vi "Assemble_Vision_Judge.vi"(11 "D3006 R合蓋結果":bool[](array[boolean])) -> (2 "結果":string)   [LabVIEW 2019]
panel:
  out "appended array":bool[](array[boolean])
  # "1. 無定位點\n2. 無塑膠件\n3. 無旋開\n4. 無限位\n5. 保留一\n6. 保留二"
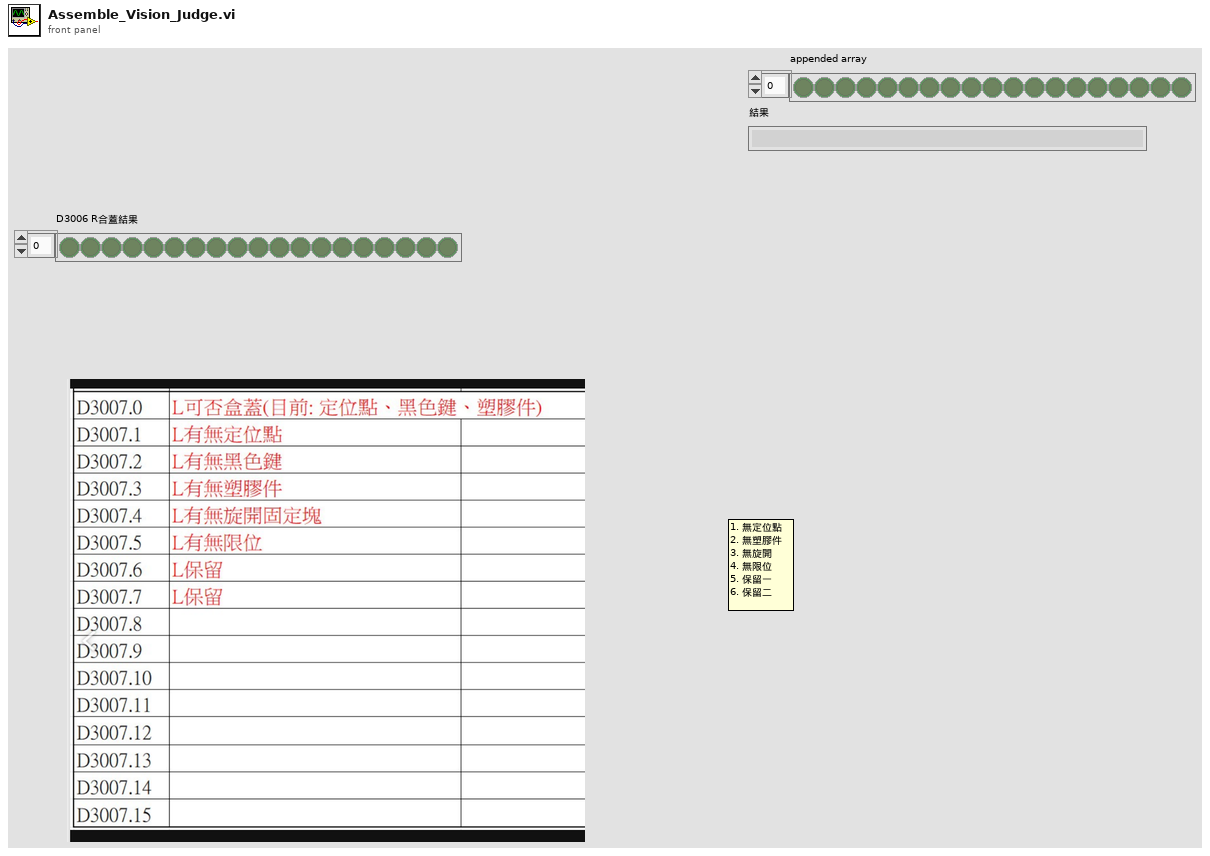
[diagram p1: front panel]
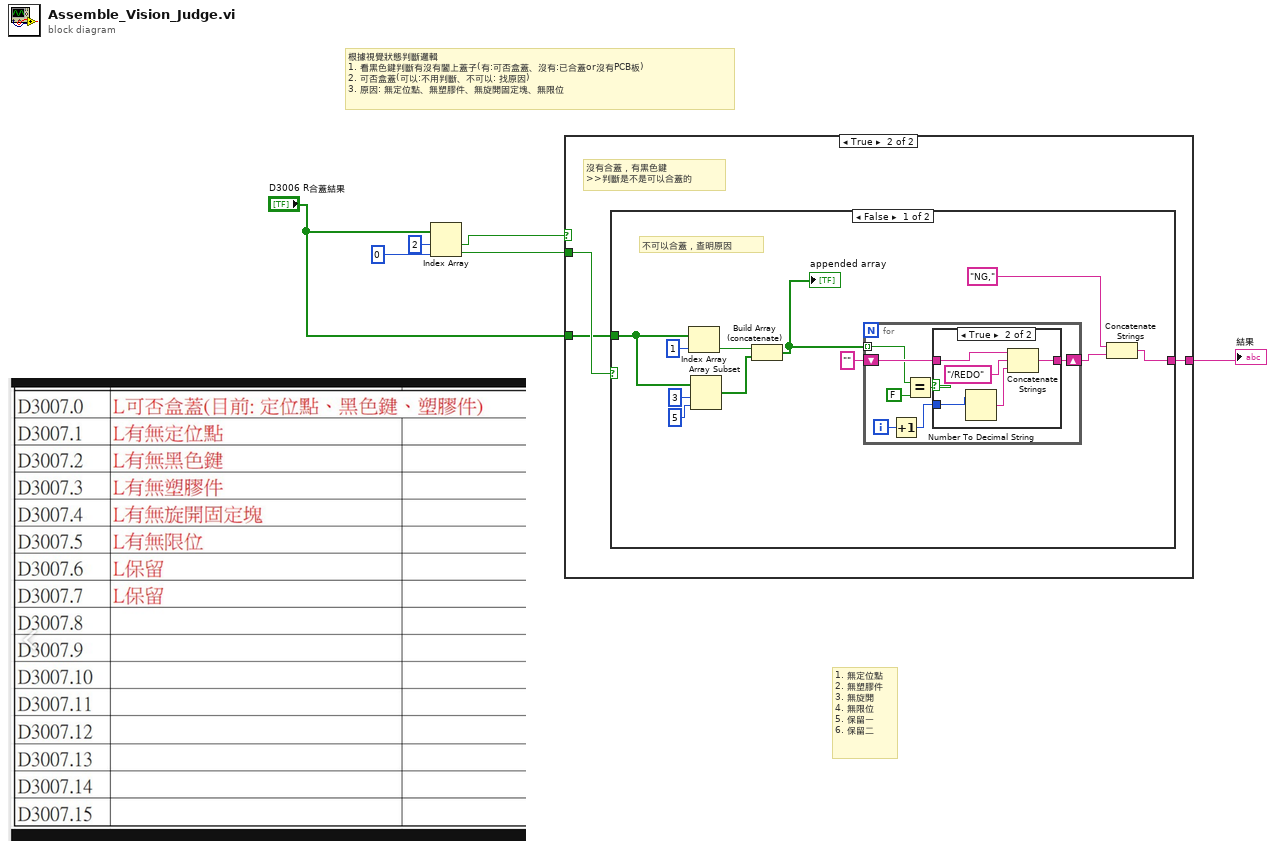
[diagram p0: block diagram]
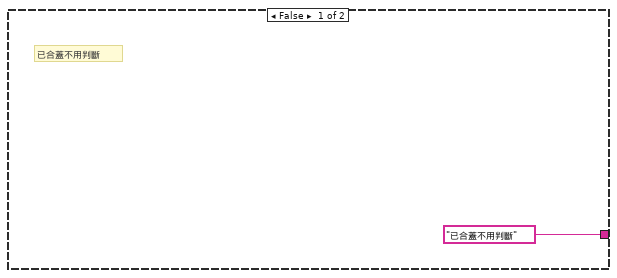
[diagram p2: hidden frame]
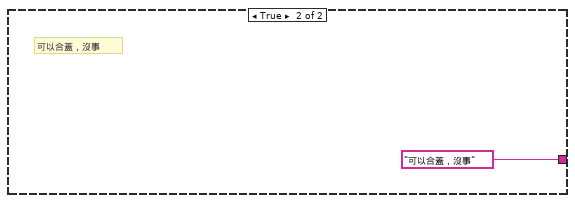
[diagram p4: hidden frame]
diagram:
  # "1. 無定位點\n2. 無塑膠件\n3. 無旋開\n4. 無限位\n5. 保留一\n6. 保留二"
  # "根據視覺狀態判斷邏輯\n1. 看黑色鍵判斷有沒有闔上蓋子(有:可否盒蓋、沒有:已合蓋or沒有PCB板)\n2. 可否盒蓋(可以:不用判斷、不可以: 找原因)\n3. 原因: 無定位點、無塑膠件、無旋開固定塊、無限位"
  n1 = Index Array(array="D3006 R合蓋結果", index #1=2 ("index"), index #2=0 ("index")) -> (element #1=w5:bool, element #2=w3:bool)
  n2 = case shown="True" w5 {
    tunnel: w3 -> [_ w10]
    tunnel: "D3006 R合蓋結果" -> [_ w9]
    tunnel: ["已合蓋不用判斷" w8] -> w1
    frame False {
      # "已合蓋不用判斷"
    }
    frame True {
      # "沒有合蓋，有黑色鍵\n>>判斷是不是可以合蓋的"
      n3 = case shown="False" w10 {
        tunnel: w9 -> [w20 _]
        tunnel: [w11 "可以合蓋，沒事"] -> w8
        frame False {
          # "不可以合蓋，查明原因"
          n4 = Index Array(array=w20, index=1) -> (element=w17:bool)
          n5 = Array Subset(array=w20, index=3, length=5) -> (w16:bool[])
          n6 = Build Array (concatenate)(w17, w16) -> (w14:bool[])
          "appended array" <- w14
          n7 = for {
            tunnel: w14 -> [w26] mode=indexing
            shift-right: [w22] -> w13
            shift-left: "" -> [w28]
            i -> [w24]
            n8 = Increment(x=w24) -> (x+1=w23:i32)
            n9 = Equal?(x=w26, y=FALSE) -> (x = y?=w25:bool)
            n10 = case shown="True" w25 {
              tunnel: w28 -> [w29 w34]
              tunnel: w23 -> [_ w32]
              tunnel: [w29 w30] -> w22
              frame False {
              }
              frame True {
                n11 = Number To Decimal String(number=w32) -> (decimal integer string=w31:string)  [unwired: 1 in]
                n12 = Concatenate Strings(w34, "/REDO" ("string"), w31) -> (w30:string)
              }
            }
          }
          n13 = Concatenate Strings("NG,", w13) -> (w11:string)
        }
        frame True {
          # "可以合蓋，沒事"
        }
      }
    }
  }
  "結果" <- w1
